vi "CAN Test.vi"() -> (0 "error out":errorcluster)   [LabVIEW 2019, in "Wrappers.lvlib"]
uses:
  Wrappers.lvlib
  CAN/Setting.ctl
  CAN/CAN.lvclass
panel:
  out "Rx out Arr":dbl[](array[numeric])=[0.0, 81.0, 77.0, 0.0, 0.0]
  in  "Rx Array SN":string[](array[string])=["GIP_Status.GIP_State", "GIP_GetSerialNumber.vendorChar0", "GIP_GetSerialNumber.vendorChar1", "GIP_GetSerialNumber.vendorChar2", "GIP_GetSerialNumber.weekAndSerial"]
  in  "Tx Signal In":string="GIP_SetSerialNumber.vendorChar1"
  in  "Signal Write":dbl=77.0
  in  "Send Tx":bool
  in  "stop":bool
  in  "Interface":refnum<k21>="CAN1"
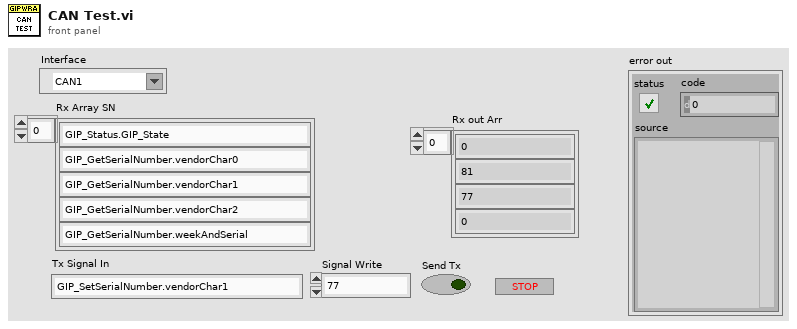
[diagram p1: front panel]
types:
  T1 = typedef "CAN.lvclass/Setting.ctl" = cluster{"Termination":u32, "Baud Rate":u64, "Interface":refnum<k21>, "XNET Database":refnum<k21>, "ECU":refnum<k21>}
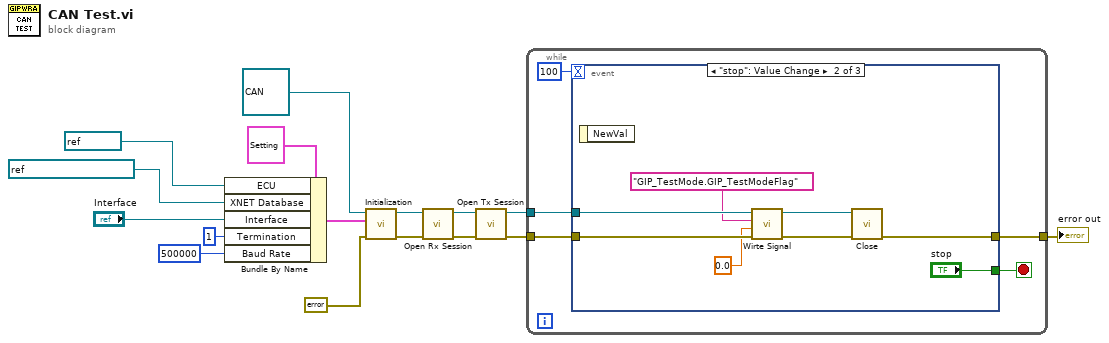
[diagram p0: block diagram]
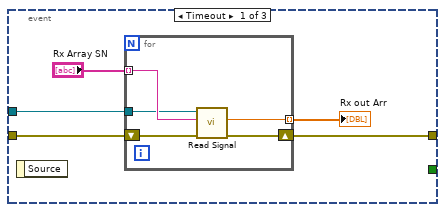
[diagram p2: hidden frame]
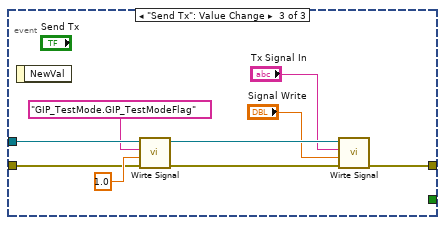
[diagram p3: hidden frame]
diagram:
  n1 = Bundle By Name(cluster=T1 {"Termination"=1, "Baud Rate"=125000, "Interface"="CAN1", "XNET Database"="GIP_CAN_Database", "ECU"="GIP\nGIP_CAN_Database"} ("Setting"), "ECU"=refnum<k21> "GIP\ncan_messages_818", "XNET Database"=refnum<k21> "can_messages_818", "Interface"="Interface", "Termination"=u32 1, "Baud Rate"=u64 500000) -> (w4:T1)
  n2 = call "Initialization.vi"("error in (no error)"=errorcluster {"status"=FALSE, "code"=0, "source"=""} ("error in"), "Setting"=w4, "CAN in"=refnum<class "CAN.lvclass"> refnum ("CAN.lvclass")) -> ("error out"=w7:errorcluster, "CAN out"=w9:refnum<class "CAN.lvclass">)  [unwired: 7 in]
  n3 = call "Open Rx Session.vi"("error in (no error)"=w7, "CAN in"=w9) -> ("error out"=w8:errorcluster, "CAN out"=w10:refnum<class "CAN.lvclass">)  [unwired: 8 in]
  n4 = call "Open Tx Session.vi"("error in (no error)"=w8, "CAN in"=w10) -> ("error out"=w5:errorcluster, "CAN out"=w1:refnum<class "CAN.lvclass">)  [unwired: 8 in]
  n5 = while {
    tunnel: [w19] -> w11
    tunnel: w5 -> [w20]
    tunnel: w1 -> [w17]
    stop <- w21 stop-if-true
    n6 = event shown="[1] \"stop\": Value Change" {
      selector: _ -> [_ _ _]
      dyn-events: _ -> [_ _ _]
      timeout: 100 -> [_ _ _]
      tunnel: [_ "stop" _] -> w21
      tunnel: w20 -> [w26 w38 w46]
      tunnel: [w25 w33 w40] -> w19
      tunnel: w17 -> [w22 w37 w48]
      event Timeout {
        n7 = event-data() -> ()  [unwired: 1 in, 1 out]
        n8 = for {
          tunnel: "Rx Array SN" -> [w28] mode=indexing
          tunnel: [w29] -> w24 mode=indexing
          shift-right: [w30] -> w25
          shift-left: w26 -> [w31]
          tunnel: w22 -> [w27]
          n9 = call "Read Signal.vi"("error in (no error)"=w31, "Rx Signal In"=w28, "CAN in"=w27) -> ("error out"=w30:errorcluster, "Signal out"=w29:dbl)  [unwired: 6 in, 1 out]
        }
        "Rx out Arr" <- w24
      }
      event "stop": Value Change {
        n10 = event-data() -> ()  [unwired: 1 in, 1 out]
        n11 = call "Wirte Signal.vi"("error in (no error)"=w38, "Signal Write"=0.0, "Tx Signal In"="GIP_TestMode.GIP_TestModeFlag", "CAN in"=w37) -> ("error out"=w34:errorcluster, "CAN out"=w32:refnum<class "CAN.lvclass">)  [unwired: 6 in]
        n12 = call "Close.vi"("error in (no error)"=w34, "CAN in"=w32) -> ("error out"=w33:errorcluster)  [unwired: 8 in, 1 out]
      }
      event "Send Tx": Value Change {
        n13 = event-data() -> ()  [unwired: 1 in, 1 out]
        n14 = call "Wirte Signal.vi"("error in (no error)"=w46, "Signal Write"=1.0, "Tx Signal In"="GIP_TestMode.GIP_TestModeFlag", "CAN in"=w48) -> ("error out"=w44:errorcluster, "CAN out"=w43:refnum<class "CAN.lvclass">)  [unwired: 6 in]
        n15 = call "Wirte Signal.vi"("error in (no error)"=w44, "Signal Write"="Signal Write", "Tx Signal In"="Tx Signal In", "CAN in"=w43) -> ("error out"=w40:errorcluster)  [unwired: 6 in, 1 out]
      }
    }
  }
  "error out" <- w11
